vi "RSZVB Check Option.vi"(8 "error in (no error)":errorcluster {"code" format="%.0x"}, 10 "Options":string, 11 "VISA session":refnum<visa-resource-name>) -> (0 "error out":errorcluster {"code" format="%.0x"}, 3 "dup VISA session":refnum<visa-resource-name>)   [LabVIEW 2015]
doc: "This VI reads data from the instrument's output buffer and returns it to the specified variable in memory.\n\nNotes:\n\n(1) Because the instrument may return both numeric and text data in response to queries this VI returns the data in string format.\n\n(2) If valid data is not available at the instrument's output buffer when this VI is called the instrument will hang up and the function will not return until it times out. If the time-out is disabled this function will hang indefinitely and it may be necessary to reboot the computer to break out."
uses:
  _utility/RSZVB Global Data.vi
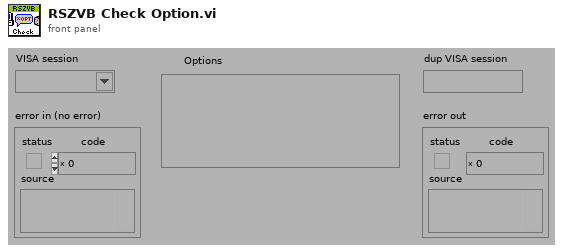
[diagram p1: front panel]
types:
  T1 = cluster{"Error Checking (T: On)":bool, "Installed Options":string[], "Data Valid?":bool, "Ports":i32, "Model":string[], "Option Checking (T: On)":bool}[]
  T2 = cluster{"Error Checking (T: On)":bool, "Installed Options":string[], "Data Valid?":bool, "Ports":i32, "Model":string[], "Option Checking (T: On)":bool}
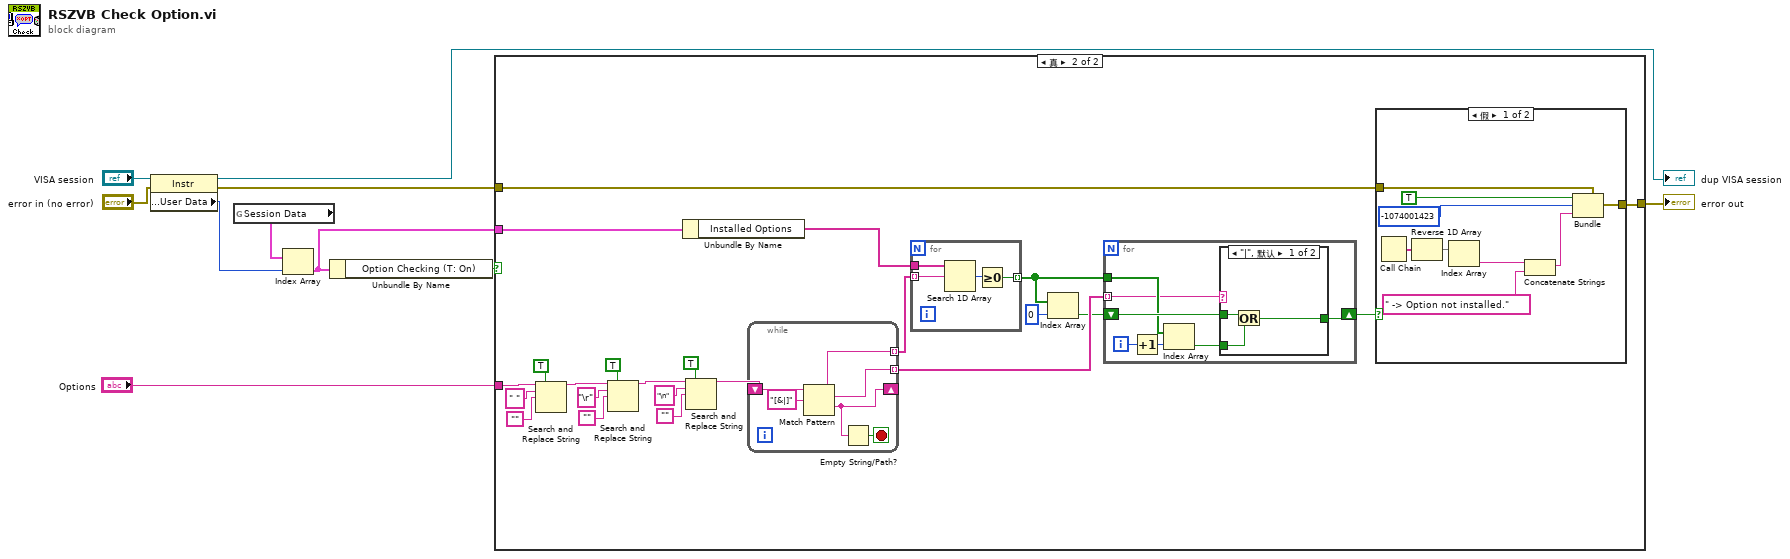
[diagram p0: block diagram]
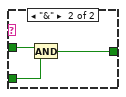
[diagram p4: hidden frame]
diagram:
  n1 = property class="Instr"(reference="VISA session", error in="error in (no error)") -> (reference out=→"dup VISA session":refnum<visa-resource-name>, error out=w7:errorcluster, "General Settings:User Data"=w8:u32)
  n2 = global read "RSZVB Global Data.vi" "Session Data"() -> (w2:T1)
  n3 = Index Array(array=w2, index=w8) -> (element=w3:T2)
  n4 = Unbundle By Name(w3) -> ("Option Checking (T: On)"=w1:bool)
  n5 = case shown="真" w1 {
    tunnel: w7 -> [w11 w22]
    tunnel: [w11 w21] -> w5
    tunnel: "Options" -> [_ w34]
    tunnel: w3 -> [_ w29]
    frame False {
    }
    frame True {
      n6 = Search and Replace String(replace all?=TRUE ("replace all? (F)"), input string=w34, search string=" ", replace string="") -> (result string=w14:string)  [unwired: 4 in, 3 out]
      n7 = Search and Replace String(replace all?=TRUE ("replace all? (F)"), input string=w14, search string="\r", replace string="") -> (result string=w13:string)  [unwired: 4 in, 3 out]
      n8 = Unbundle By Name(w29) -> ("Installed Options"=w28:string[])
      n9 = Search and Replace String(replace all?=TRUE ("replace all? (F)"), input string=w13, search string="\n", replace string="") -> (result string=w12:string)  [unwired: 4 in, 3 out]
      n10 = while {
        shift-right: [w65] -> _
        shift-left: w12 -> [w67]
        tunnel: [w64] -> w30 mode=indexing
        tunnel: [w63] -> w27 mode=indexing
        stop <- w62 stop-if-true
        n11 = Match Pattern(string=w67, regular expression="[&|]") -> (before substring=w64:string, match substring=w63:string, after substring=w65:string)  [unwired: 1 in, 1 out]
        n12 = Empty String/Path?(string/path=w65) -> (empty?=w62:bool)
      }
      n13 = for {
        tunnel: w30 -> [w61] mode=indexing
        tunnel: w28 -> [w60]
        tunnel: [w58] -> w25 mode=indexing
        n14 = Search 1D Array(1D array=w60, element=w61) -> (index of element=w59:i32)  [unwired: 1 in]
        n15 = Greater Or Equal To 0?(x=w59) -> (x >= 0?=w58:bool)
      }
      n16 = Index Array(array=w25, index=0) -> (element=w26:bool)
      n17 = for {
        tunnel: w27 -> [w45] mode=indexing
        tunnel: w25 -> [w49]
        shift-right: [w50] -> w23
        shift-left: w26 -> [w51]
        i -> [w47]
        n18 = Increment(x=w47) -> (x+1=w48:i32)
        n19 = Index Array(array=w49, index=w48) -> (element=w46:bool)
        n20 = case shown="\"|\", 默认" w45 {
          tunnel: w51 -> [w53 w57]
          tunnel: [w54 w56] -> w50
          tunnel: w46 -> [w52 w55]
          frame "|", Default {
            n21 = Or(x=w53, y=w52) -> (x .or. y?=w54:bool)
          }
          frame "&" {
            n22 = And(x=w57, y=w55) -> (x .and. y?=w56:bool)
          }
        }
      }
      n23 = case shown="假" w23 {
        tunnel: w22 -> [w43 w44]
        tunnel: [w41 w44] -> w21
        frame False {
          n24 = Call Chain() -> (call chain=w39:string[])
          n25 = Reverse 1D Array(array=w39) -> (reversed array=w38:string[])
          n26 = Index Array(array=w38) -> (element=w37:string)  [unwired: 1 in]
          n27 = Concatenate Strings(w37, " -> Option not installed." ("string")) -> (w35:string)
          n28 = Bundle(cluster=w43, "status"=TRUE, "code"=-1074001423, "source"=w35) -> (w41:errorcluster)
        }
        frame True {
        }
      }
    }
  }
  "error out" <- w5
